vi "Build_Cluster_HGB2_Rev01.vi"() -> (3 "output cluster":T1)   [LabVIEW 2016]
panel:
  in  "On/Off":dbl
  in  "Speed Setpoint":dbl
  in  "NI 6001":waveform(dbl)[](array[waveform])
  in  "Operator Notes":string
  in  "Dummy Variable":dbl
  in  "Accelerometer":waveform(dbl)[](array[waveform])
  in  "Data Main":waveform(dbl)[](array[waveform])
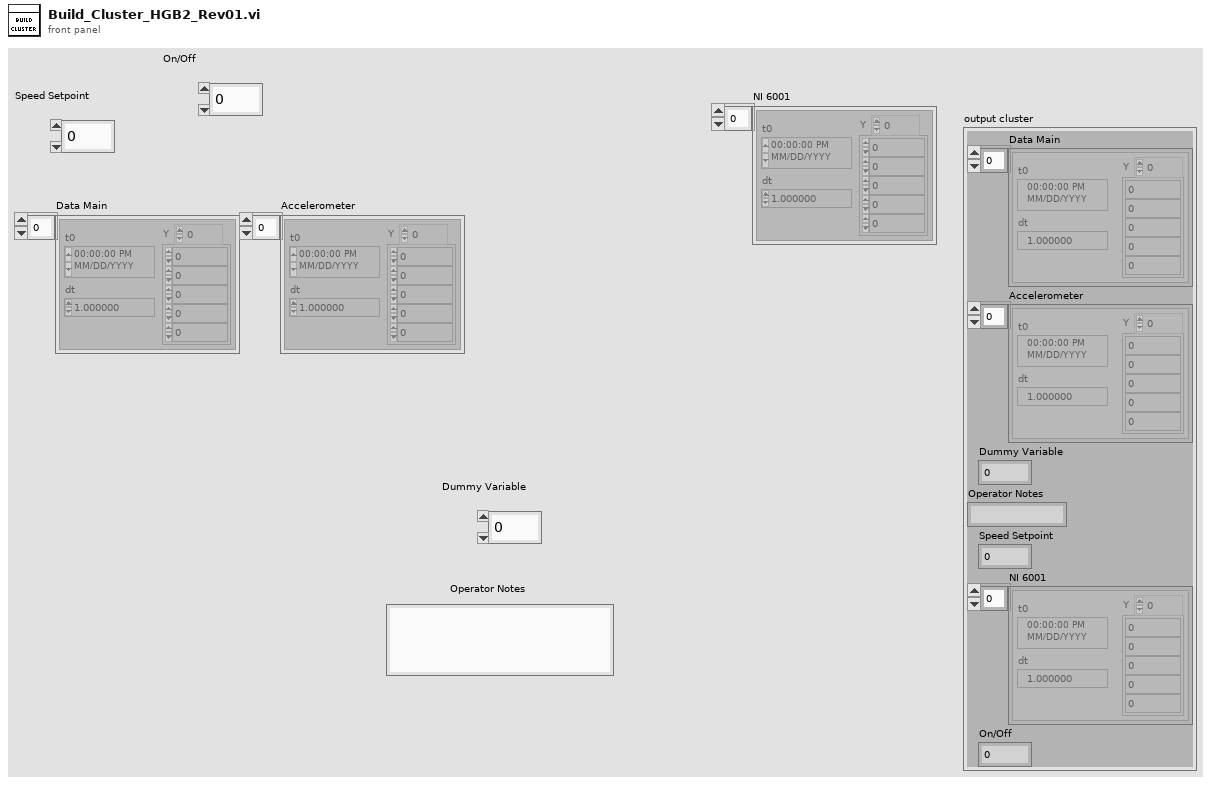
[diagram p1: front panel]
types:
  T1 = cluster{"Data Main":waveform(dbl)[], "Accelerometer":waveform(dbl)[], "Dummy Variable":dbl, "Operator Notes":string, "Speed Setpoint":dbl, "NI 6001":waveform(dbl)[], "On/Off":dbl}
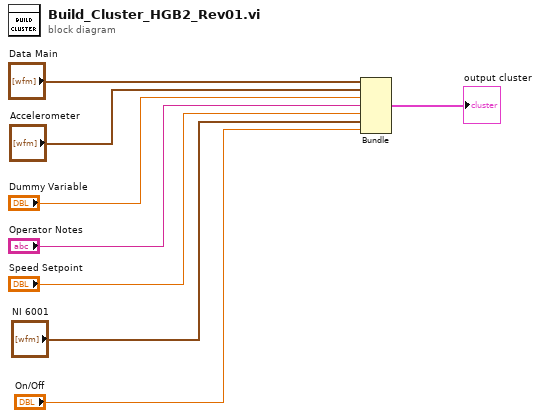
[diagram p0: block diagram]
diagram:
  n1 = Bundle("Data Main"="Data Main", "Accelerometer"="Accelerometer", "Dummy Variable"="Dummy Variable", "Operator Notes"="Operator Notes", "Speed Setpoint"="Speed Setpoint", "NI 6001"="NI 6001", "On/Off"="On/Off") -> (→"output cluster":T1)  [unwired: 1 in]
